vi "VG_EquipementsNeeded.vi"() -> ()   [LabVIEW 2020]
panel:
  out "VG_EquipementsNeeded":string[](array[string])
  # "Dans le fichier de config, les equipements doit etre identifié dans cet ordre"
  # "ITECH\n\nHIOKI ST5520\n\nTENMA\n\nBT3564"
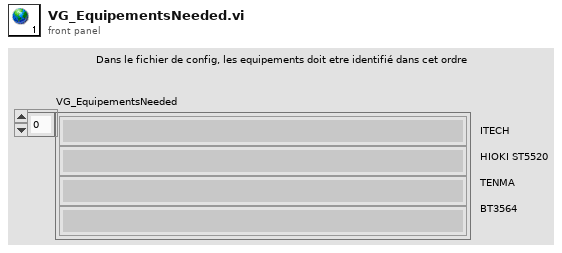
[diagram p1: front panel]
diagram:
